vi "shift-arraysSD.vi"(2 "in2":dbl[](array[numeric]), 3 "inverted":bool, 4 "in1":dbl[](array[numeric])) -> (0 "out2":dbl[](array[numeric]), 1 "out1":dbl[](array[numeric]))   [LabVIEW 2015]
uses:
  globalVarSD.vi
panel:
  out "Graphe 4":dbl[](graph)
  out "Graphe 3":dbl[](graph)
  out "Graphe 2":dbl[](graph)
  out "Graphe":dbl[](graph)
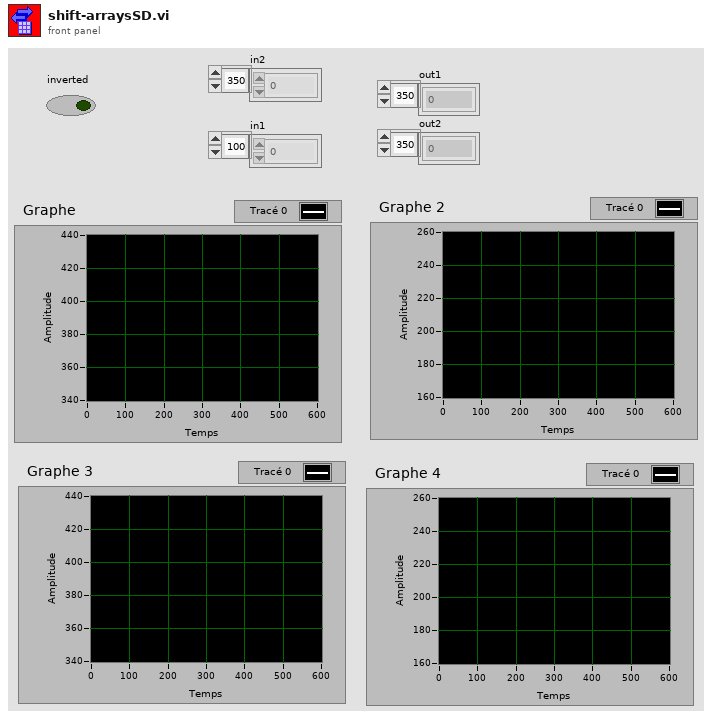
[diagram p1: front panel]
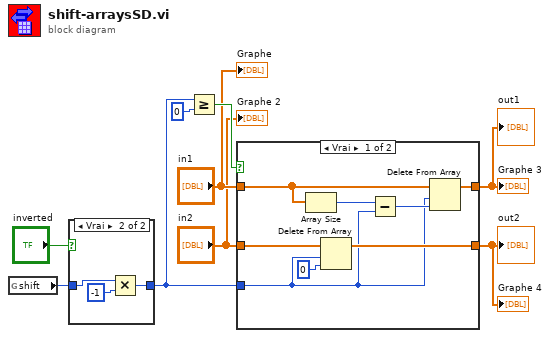
[diagram p0: block diagram]
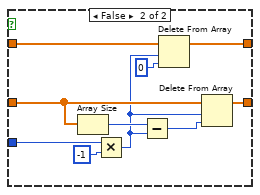
[diagram p3: hidden frame]
diagram:
  n1 = global read "globalVarSD.vi" "shift"() -> (w6:i32)
  n2 = case shown="Vrai" "inverted" {
    tunnel: [w10 w11] -> w5
    tunnel: w6 -> [w10 w13]
    frame False {
    }
    frame True {
      n3 = Multiply(x=w13, y=-1 ("x")) -> (x*y=w11:i32)
    }
  }
  n4 = Greater Or Equal?(x=w5, y=0) -> (x >= y?=w9:bool)
  n5 = case shown="Vrai" w9 {
    tunnel: "in1" -> [w21 w26]
    tunnel: w5 -> [w15 w29]
    tunnel: "in2" -> [w18 w27]
    tunnel: [w17 w24] -> w2
    tunnel: [w16 w25] -> w1
    frame True {
      n6 = Array Size(array=w21) -> (size(s)=w20:i32)
      n7 = Delete From Array(array=w18, length=w15, index=0) -> (array with subset deleted=w16:dbl[])  [unwired: 1 out]
      n8 = Subtract(x=w20, y=w15) -> (x-y=w19:i32)
      n9 = Delete From Array(array=w21, length=w15, index=w19) -> (array with subset deleted=w17:dbl[])  [unwired: 1 out]
    }
    frame False {
      n10 = Array Size(array=w27) -> (size(s)=w31:i32)
      n11 = Multiply(x=w29, y=-1) -> (x*y=w23:i32)
      n12 = Subtract(x=w31, y=w23) -> (x-y=w30:i32)
      n13 = Delete From Array(array=w26, length=w23, index=0) -> (array with subset deleted=w24:dbl[])  [unwired: 1 out]
      n14 = Delete From Array(array=w27, length=w23, index=w30) -> (array with subset deleted=w25:dbl[])  [unwired: 1 out]
    }
  }
  "out1" <- w2
  "out2" <- w1
  "Graphe 3" <- w2
  "Graphe 4" <- w1
  "Graphe" <- "in1"
  "Graphe 2" <- "in2"
